vi "reset.vi"(8 "error in (no error)":errorcluster, 11 "GenericSignalReader in":refnum<class "GenericSignalReader.lvclass">) -> (0 "error out":errorcluster, 3 "GenericSignalReader out":refnum<class "GenericSignalReader.lvclass">)   [LabVIEW 2010, in "GenericSignalReader.lvclass"]
uses:
  GenericSignalReader.lvclass
  GenericSignalReader.lvclass/GenericSignalReader.ctl
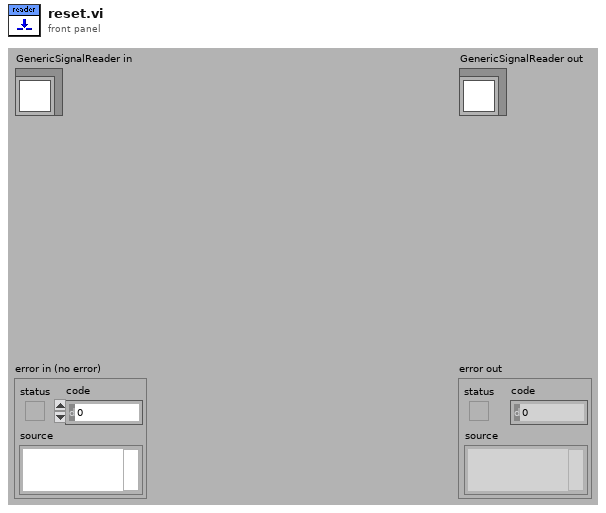
[diagram p1: front panel]
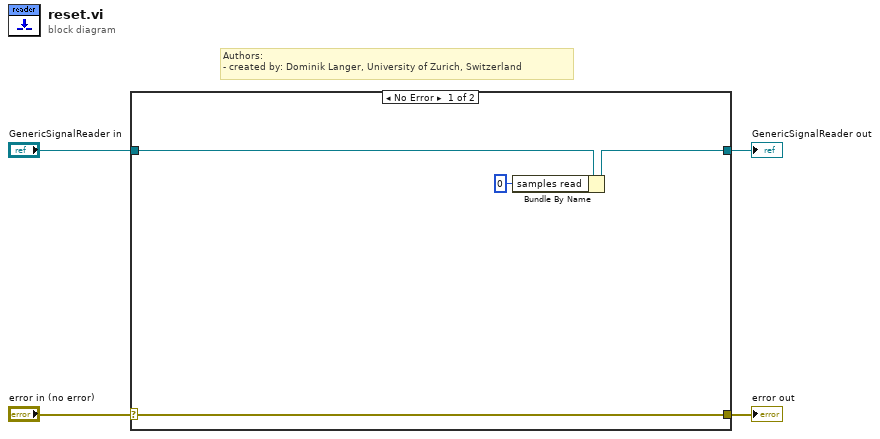
[diagram p0: block diagram]
diagram:
  # "Authors: \n- created by: Dominik Langer, University of Zurich, Switzerland"
  n1 = case shown="No Error" "error in (no error)" {
    selector: "error in (no error)" -> [w8 w10]
    tunnel: [w8 w10] -> w3
    tunnel: [w5 w9] -> w1
    tunnel: "GenericSignalReader in" -> [w6 w9]
    frame No Error {
      n2 = Bundle By Name(cluster=w6, "samples read"=0) -> (w5:refnum<class "GenericSignalReader.lvclass">)
    }
    frame Error {
    }
  }
  "error out" <- w3
  "GenericSignalReader out" <- w1
